vi "Back.vi"() -> ()   [LabVIEW 2021]
uses:
  Demo_server/RPC Service/Communicate/Communicate.lvclass
  <vilib>/gRPC/LabVIEW gRPC Library/Shared/grpcId.ctl
  <vilib>/gRPC/LabVIEW gRPC Servicer/Servicer/Servicer.lvclass/Servicer.ctl
  Demo_server/RPC Service/Communicate/Communicate.lvclass/Communicate.ctl
  Demo_server/RPC Messages/Communication_StreamData.ctl
  <vilib>/gRPC/LabVIEW gRPC Servicer/Servicer/Servicer.lvclass
  Demo_server/Demo_server.lvlib
  <vilib>/gRPC/LabVIEW gRPC Library/grpc-lvsupport-release.lvlib
panel:
  out "Running?":bool
  out "Listening Port":i32
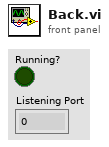
[diagram p1: front panel]
types:
  T1 = typedef "grpc-lvsupport-release.lvlib/grpcId.ctl" = u64
  T2 = cluster{"Running?":bool, "gRPCid out":T1, "Index":i32}
  T3 = typedef "Demo_server.lvlib/Communicate.lvclass/Server gRPC UEs.ctl" = cluster{"Communicate Stream gRPC UE":refnum<user-event>}
  T4 = typedef "Demo_server.lvlib/Communication_StreamData.ctl" = cluster{"data":i32, "Status":bool}
  T5 = typedef "Demo_server.lvlib/Communication_ControlStream.ctl" = cluster{"Start":bool}
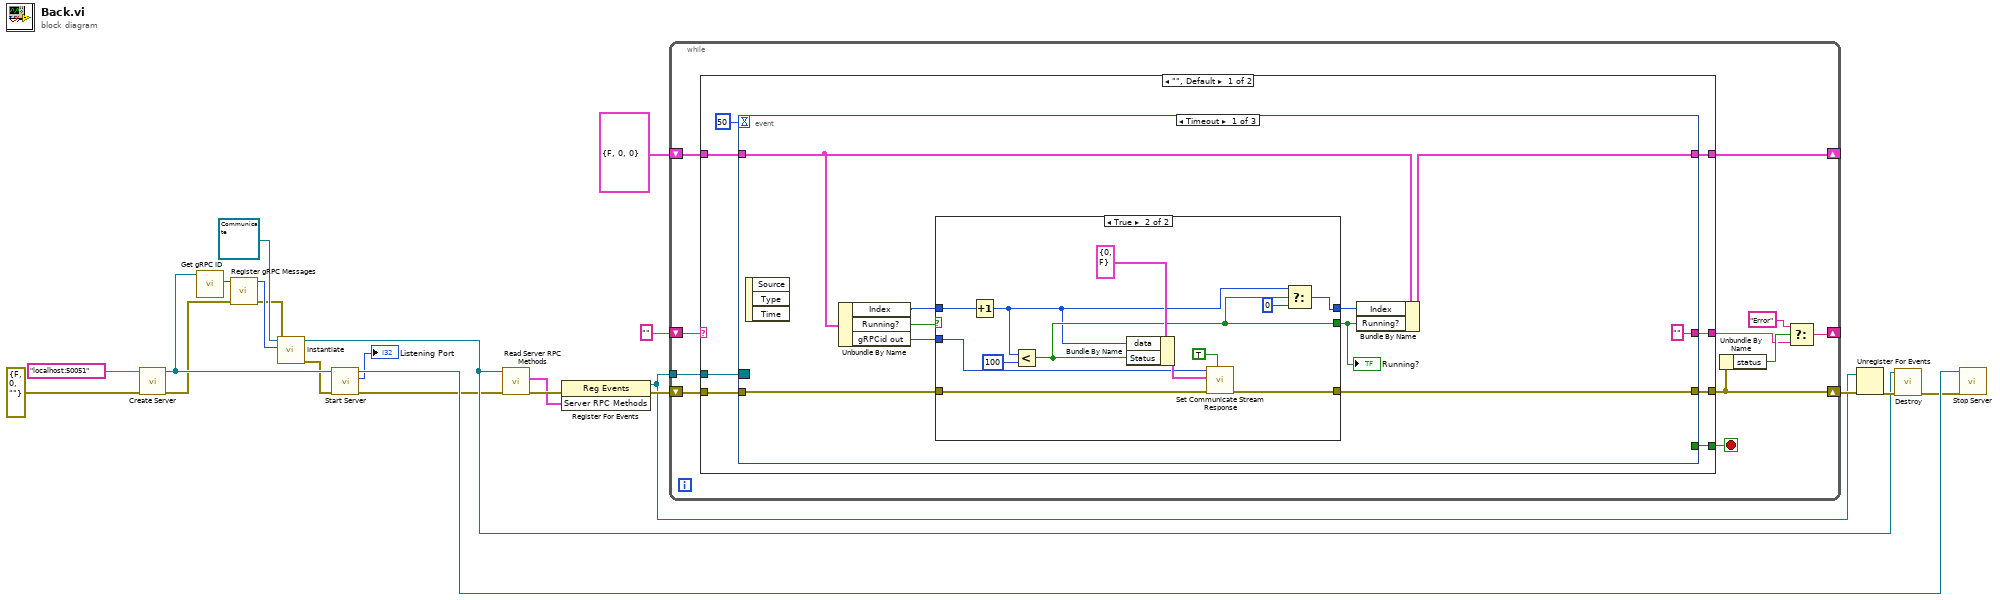
[diagram p0: block diagram]
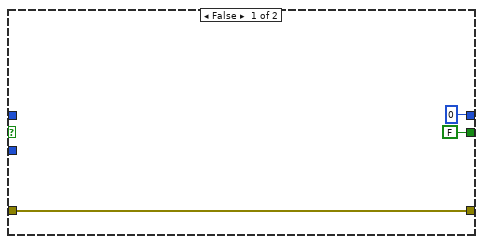
[diagram p2: hidden frame]
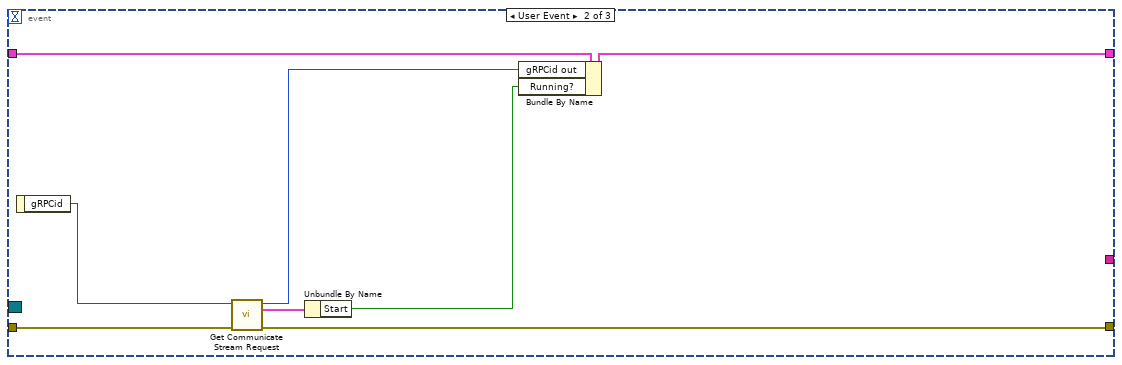
[diagram p3: hidden frame]
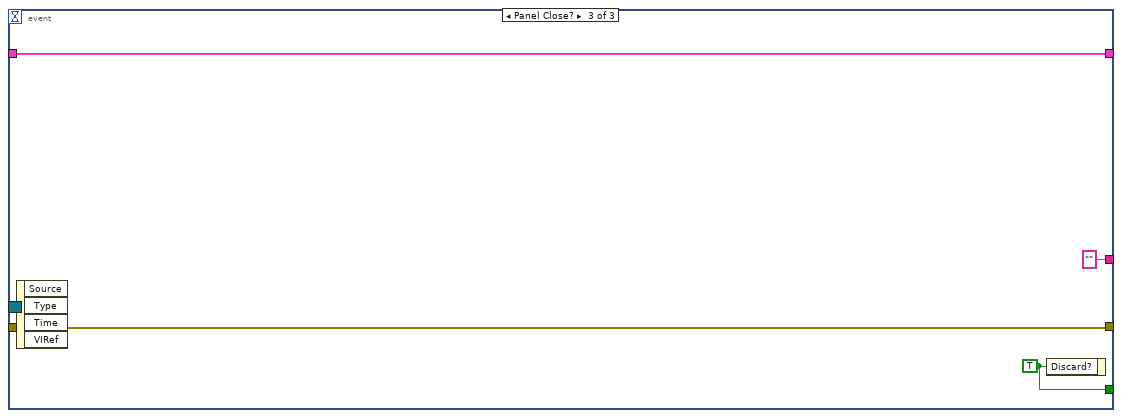
[diagram p4: hidden frame]
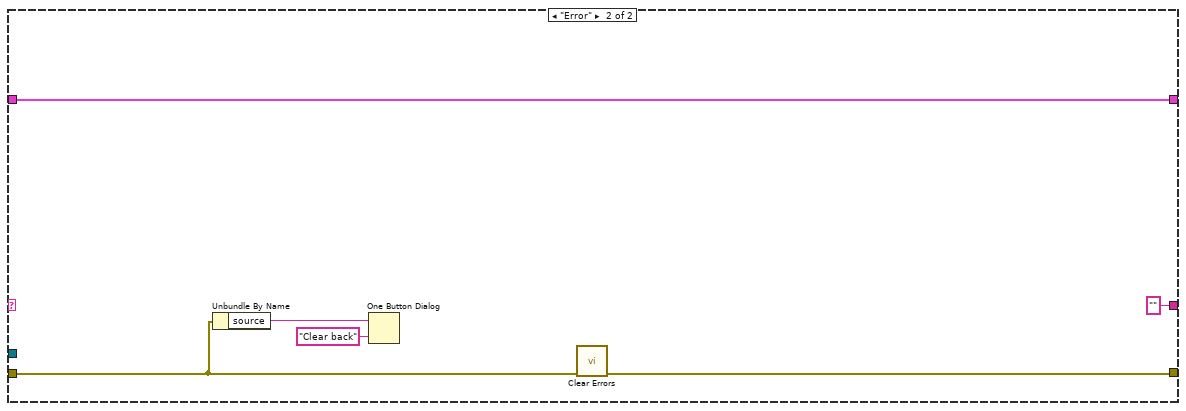
[diagram p5: hidden frame]
diagram:
  n1 = call <vilib>:"Create Server.vi"("error in"=errorcluster {"status"=FALSE, "code"=0, "source"=""} ("error in (no error)"), "Server Address"="localhost:50051") -> ("error out"=w3:errorcluster, "gRPC Server out"=w14:refnum<class "Servicer.lvclass">)  [unwired: 8 in]
  n2 = call <vilib>:"Get gRPC ID.vi"("OOP Server in"=w14) -> ("gRPC ID"=w4:T1)  [unwired: 9 in, 1 out]
  n3 = call "Register gRPC Messages.vi"("error in (no error)"=w3, "gRPC ID"=w4) -> ("error out"=w2:errorcluster, "gRPC ID Out"=w5:T1)  [unwired: 8 in]
  n4 = call-dynamic "Instantiate.vi"("error in"=w2, "gRPCid"=w5, "iService"=refnum<class "Communicate.lvclass"> refnum ("gRPC Server in")) -> ("error out"=w13:errorcluster, "iService"=w7:refnum<class "Communicate.lvclass">)  [unwired: 7 in]
  n5 = call <vilib>:"Start Server.vi"("error in"=w13, "gRPC Server in"=w14) -> ("error out"=w6:errorcluster, "Listening Port"=→"Listening Port":i32, "gRPC Server out"=w16:refnum<class "Servicer.lvclass">)  [unwired: 7 in]
  n6 = call "Read Server RPC Methods.vi"("error in (no error)"=w6, "SignalGeneratorService in"=w7) -> ("error out"=w9:errorcluster, "Server RPC Methods"=w8:T3)  [unwired: 7 in, 1 out]
  n7 = register-events(error in=w9, w8) -> (reference out=w19:refnum<event-registration>, error out=w21:errorcluster)  [unwired: 1 in]
  n8 = while {
    shift-right: [w30] -> w20
    shift-left: w21 -> [w32]
    shift-right: [w28] -> _
    shift-left: "" -> [w33]
    tunnel: w19 -> [w25]
    shift-right: [w23] -> _
    shift-left: T2 {"Running?"=FALSE, "gRPCid out"=0, "Index"=0} -> [w24]
    stop <- w31 stop-if-true
    n9 = case shown="\"\", Default" w33 {
      tunnel: w32 -> [w41 w83]
      tunnel: [w40 w84] -> w30
      tunnel: [w39 ""] -> w27
      tunnel: [w38 _] -> w31
      tunnel: w25 -> [w36 _]
      tunnel: w24 -> [w35 w79]
      tunnel: [w34 w79] -> w23
      frame "", Default {
        n10 = event shown="[0] Timeout" {
          selector: w36 -> [_ _ _]
          dyn-events: _ -> [_ _ _]
          timeout: 50 -> [_ _ _]
          tunnel: w41 -> [w49 w72 w78]
          tunnel: [w50 w71 w78] -> w40
          tunnel: ["" _ ""] -> w39
          tunnel: [_ _ w76] -> w38
          tunnel: w35 -> [w48 w74 w75]
          tunnel: [w45 w70 w75] -> w34
          event Timeout {
            n11 = event-data() -> ()  [unwired: 1 in, 3 out]
            n12 = Unbundle By Name(w48) -> ("Index"=w46:i32, "Running?"=w42:bool, "gRPCid out"=w47:T1)
            n13 = case shown="True" w42 {
              tunnel: [w54 w66] -> w50
              tunnel: w49 -> [w54 w65]
              tunnel: w47 -> [_ w61]
              tunnel: w46 -> [_ w60]
              tunnel: [0 w56] -> w44
              tunnel: [FALSE w58] -> w43
              frame False {
              }
              frame True {
                n14 = Increment(x=w60) -> (x+1=w57:i32)
                n15 = Less?(x=w57, y=100) -> (x < y?=w58:bool)
                n16 = Bundle By Name(cluster=T4 {"data"=0, "Status"=FALSE} ("Message Data"), "data"=w57, "Status"=w58) -> (w63:T4)
                n17 = call "Set Communicate Stream Response.vi"("Streaming? (F)"=TRUE, "error in (no error)"=w65, "Message Data"=w63, "gRPCid in"=w61) -> ("error out"=w66:errorcluster)  [unwired: 7 in]
                n18 = Select(t=w57, s=w58, f=0) -> (s? t:f=w56:i32)
              }
            }
            "Running?" <- w43
            n19 = Bundle By Name(cluster=w48, "Index"=w44, "Running?"=w43) -> (w45:T2)
          }
          event User Event {
            n20 = event-data() -> ("gRPCid"=w73:T1)  [unwired: 1 in]
            n21 = call "Get Communicate Stream Request.vi"("error in (no error)"=w72, "gRPCid in"=w73) -> ("error out"=w71:errorcluster, "Message Data"=w68:T5, "gRPCid out"=w69:T1)  [unwired: 7 in]
            n22 = Unbundle By Name(w68) -> ("Start"=w67:bool)
            n23 = Bundle By Name(cluster=w74, "gRPCid out"=w69, "Running?"=w67) -> (w70:T2)
          }
          event Panel Close? {
            w76 = TRUE ("Discard?")
            n24 = event-data() -> ()  [unwired: 1 in, 4 out]
            n25 = event-data("Discard?"=w76) -> ()  [unwired: 1 in, 1 out]
          }
        }
      }
      frame "Error" {
        n26 = Unbundle By Name(w83) -> ("source"=w81:string)
        n27 = One Button Dialog(message=w81, button name ("OK")="Clear back") -> ()  [unwired: 1 out]
        n28 = call <vilib>:"Clear Errors.vi"("error in (no error)"=w83) -> ("error out"=w84:errorcluster)  [unwired: 5 in, 1 out]
      }
    }
    n29 = Unbundle By Name(w30) -> ("status"=w29:bool)
    n30 = Select(t="Error", s=w29, f=w27) -> (s? t:f=w28:string)
  }
  n31 = Unregister For Events(event registration refnum=w19, error in=w20) -> (error out=w11:errorcluster)
  n32 = call-dynamic "Destroy.vi"("error in (no error)"=w11, "SignalGeneratorService in"=w7) -> ("error out"=w12:errorcluster)  [unwired: 8 in, 1 out]
  n33 = call <vilib>:"Stop Server.vi"("error in"=w12, "gRPC Server in"=w16) -> ()  [unwired: 9 in, 1 out]
